vi "Initialize monovu subvis.vi"(7 "auto detect":bool=TRUE, 9 "platform":u16(ring) items=["Mac", "PC"], 10 "VIs to be initialized":T1(array[cluster])=[{"VI name"="SetField_popup.vi", "Control name"="platform", "Parameter"=0.0}, {"VI name"="SetTemp_popup.vi", "Control name"="platform", "Parameter"=0.0}, {"VI name"="SetStart_popup.vi", "Control name"="platform", "Parameter"=0.0}, {"VI name"="SetWaitForTemp_popup.vi", "Control name"="platform", "Parameter"=0.0}, {"VI name"="SetRemarks_popup.vi", "Control name"="platform", "Parameter"=0.0}, {"VI name"="SetRunVI_popup.vi", "Control name"="platform", "Parameter"=0.0}, {"VI name"="SetAbortVI_popup.vi", "Control name"="platform", "Parameter"=0.0}, {"VI name"="SetDevice_popup.vi", "Control name"="platform", "Parameter"=0.0}, {"VI name"="SetWaitFor_popup.vi", "Control name"="platform", "Parameter"=0.0}, {"VI name"="SetParameter_popup.vi", "Control name"="platform", "Parameter"=0.0}, {"VI name"="SetWaitForAnyVI_popup.vi", "Control name"="platform", "Parameter"=0.0}, {"VI name"="WriteVISA_popup.vi", "Control name"="platform", "Parameter"=0.0}, {"VI name"="write to log file.vi", "Control name"="platform", "Parameter"=0.0}], 11 "port number":u16=3374) -> (2 "platform used":u16(ring) items=["Mac", "PC"], 3 "port used":u16=3374)   [LabVIEW 2020]
panel:
  # "Change platform or version dependent parameters.\n1. Port depends on the the system OS and the version of the remote computer.\n2. platform (Mac or PC) affect the key mapping and the file path structure."
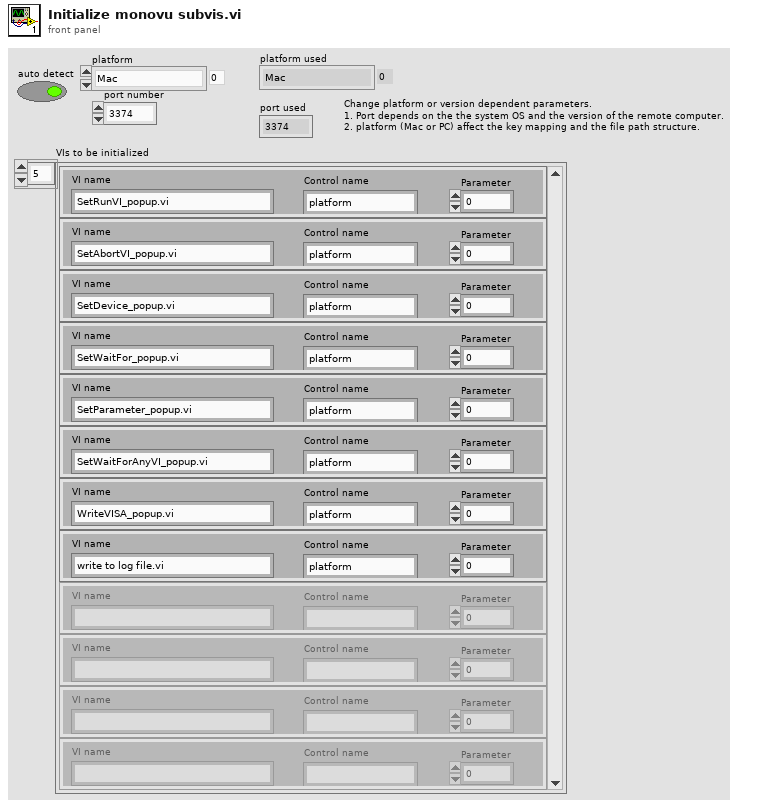
[diagram p1: front panel]
types:
  T1 = cluster{"VI name":string, "Control name":string, "Parameter":dbl}[]
  T2 = cluster{"VI name":string, "Control name":string, "Parameter":dbl}
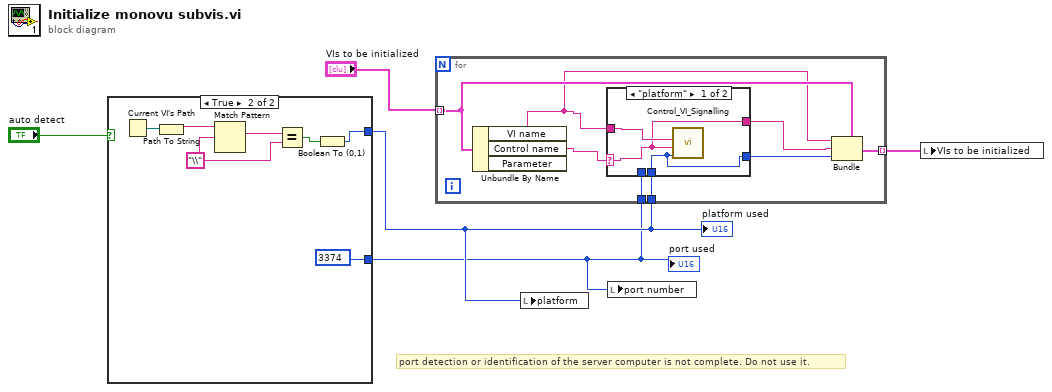
[diagram p0: block diagram]
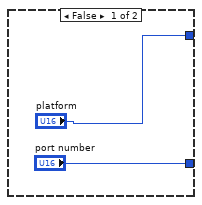
[diagram p2: hidden frame]
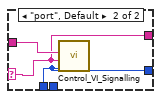
[diagram p3: hidden frame]
diagram:
  # "port detection or identification of the server computer is not complete. Do not use it."
  n1 = case shown="True" "auto detect" {
    tunnel: ["platform" w9] -> w4
    tunnel: ["port number" u16 3374 ("port number")] -> w3
    frame False {
    }
    frame True {
      w13 = "\\" ("regular expression")
      n2 = Current VI's Path() -> (path=w10:path)
      n3 = Path To String(path=w10) -> (string=w12:string)
      n4 = Match Pattern(string=w12, regular expression=w13) -> (match substring=w14:string)  [unwired: 4 out]
      n5 = Equal?(x=w14, y=w13) -> (x = y?=w11:bool)
      n6 = Boolean To (0,1)(Boolean=w11) -> (0, 1=w9:i16)
    }
  }
  "platform used" <- w4
  "port used" <- w3
  n7 = for {
    tunnel: "VIs to be initialized" -> [w19] mode=indexing
    tunnel: w4 -> [w21]
    tunnel: w3 -> [w20]
    tunnel: [w15] -> w1 mode=indexing
    n8 = Unbundle By Name(w19) -> ("VI name"=w18:string, "Control name"=w22:string)  [unwired: 1 out]
    n9 = case shown="\"platform\"" w22 {
      selector: w22 -> [w24 w27]
      tunnel: w18 -> [w25 w28]
      tunnel: w21 -> [w23 _]
      tunnel: w20 -> [_ w26]
      tunnel: [w24 w27] -> w17
      tunnel: [w23 w26] -> w16
      frame "platform" {
        n10 = call "Control_VI_Signalling.vi"("Input Value"=w23, "Control Name"=w24, "Target VI name"=w25) -> ()  [unwired: 8 in, 1 out]
      }
      frame "port", Default {
        n11 = call "Control_VI_Signalling.vi"("Input Value"=w26, "Control Name"=w27, "Target VI name"=w28) -> ()  [unwired: 8 in, 1 out]
      }
    }
    n12 = Bundle(cluster=w19, "VI name"=w18, "Control name"=w17, "Parameter"=w16) -> (w15:T2)
  }
  n13 = local write "platform"(w4) -> ()
  n14 = local write "port number"(w3) -> ()
  n15 = local write "VIs to be initialized"(w1) -> ()
